vi "FA_ApplyTDC.vi"(8 "Error In":errorcluster) -> (0 "Error Out":errorcluster)   [LabVIEW 2014, in "FA_TDC.lvlib"]
doc: "Applies the TDC config (no functionality)"
uses:
  FA_TDC.lvlib
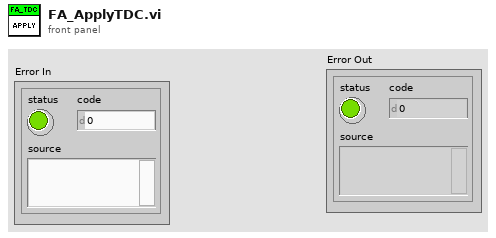
[diagram p1: front panel]
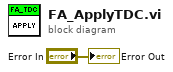
[diagram p0: block diagram]
diagram:
  "Error Out" <- "Error In"
